vi "ResultsGui.FindFiles.vi"(6 "File content prev":T1[](array[typedef]), 7 "File list tree":refnum<vi>, 8 "error in (no error)":errorcluster, 9 "PageSize (100)":i32=100, 10 "PageIdx":i32, 11 "Paths":path[](array[path])) -> (0 "error out":errorcluster, 2 "File content":T1[](array[typedef]), 3 "TotalSize":i32)   [LabVIEW 2016]
uses:
  Logger/Logger.File.ctl
  Logger/Logger.File.Properties.ctl
  Sequence/Sequence.Code.SerialFormat.ctl
  Sequence/Sequence.Counters.ctl
  Logger/Logger.File.Serials.ctl
  Sequence/Sequence.Step.Status.ctl
  <vilib>/Utility/miscctls.llb/LVRowAndColumnTypeDef.ctl
  <vilib>/Utility/miscctls.llb/LVNodeAndColumnTypeDef.ctl
  tools/Translator/Translator.Message.ctl
  tools/Translator/Translator.FormatMessage.vi
  tools/Translator/Translator.Global.vi
  Global/ApplicationGlobal.vi
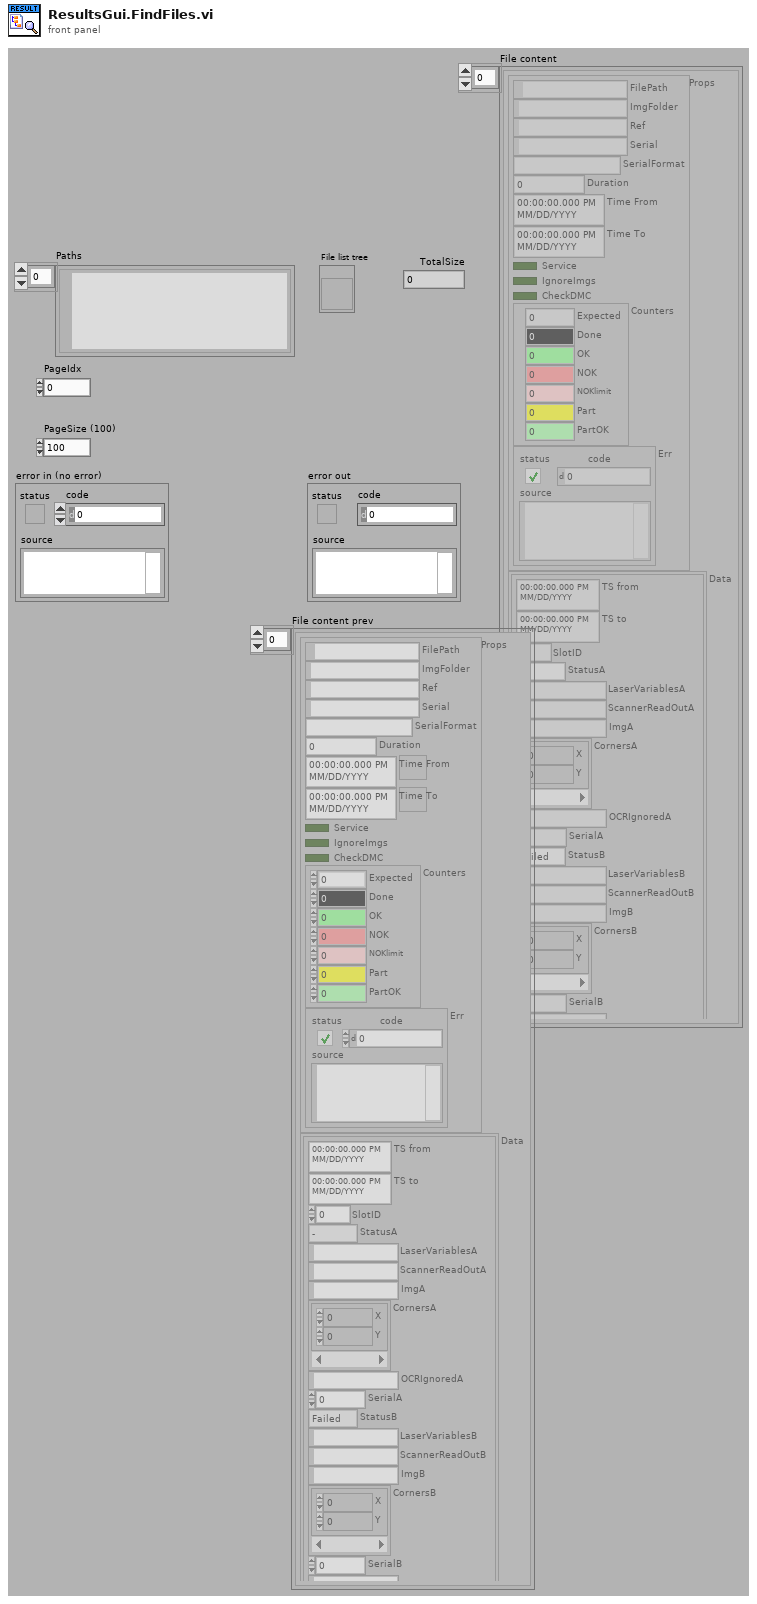
[diagram p1: front panel]
types:
  T1 = typedef "Logger.File.ctl" = cluster{"Props":T2, "Data":T5[]}
  T2 = typedef "Logger.File.Properties.ctl" = cluster{"FilePath":path, "ImgFolder":string, "Ref":string, "Serial":string, "SerialFormat":T3, "Duration":dbl, "Time From":timestamp, "Time To":timestamp, "Service":bool, "IgnoreImgs":bool, "CheckDMC":bool, "Counters":T4, "Err":errorcluster}
  T3 = typedef "Sequence.Code.SerialFormat.ctl" = enum8{"", "6 dig", "7 dig"}
  T4 = typedef "Sequence.Counters.ctl" = cluster{"Expected":u16, "Done":u16, "OK":u16, "NOK":u16, "NOKlimit":u16, "Part":u16, "PartOK":u16}
  T5 = typedef "Logger.File.Serials.ctl" = cluster{"TS from":timestamp, "TS to":timestamp, "SlotID":u8, "StatusA":T6, "LaserVariablesA":string, "ScannerReadOutA":string, "ImgA":string, "CornersA":cluster{"X":i32, "Y":i32}[], "OCRIgnoredA":string, "SerialA":u8, "StatusB":T6, "LaserVariablesB":string, "ScannerReadOutB":string, "ImgB":string, "CornersB":cluster{"X":i32, "Y":i32}[], "SerialB":u8, "OCRIgnoredB":string}
  T6 = typedef "Sequence.Step.Status.ctl" = enum16{"-", "Pending", "Running", "Skipped", "Passed", "Failed", "Done", "Error", "Aborted", "Stopped"}
  T7 = typedef "Translator.Message.ctl" = enum16{"-", "Event confirmed", "Log out", "Log in", "Shutdown", "Cancel", "Start", "Begin time", "End time", "Duration", "Service Mode", "Ignore Results", "Serial Format", "On", "Off", "OK", "NOK", "NOK %s", "Home", "Work", "Close", "Open", "In progress...", "Missing", "Empty", "Hardware failure", "Initial", "Default", "Total", "Out of range", "Free disk space is below 1GB - contact technician", "Error %d >> %s", "Error %d >> %s >> %s", "Msg %d >> %s", "Laser msg %d %s", "Laser cmd error %s %d", "Laser cmd failed %s", "Laser cmd warning %s", "Laser disconnected", "Laser status %s", "Laser already started", "Laser job unkonwn %s", "Laser job missing %s", "Laser job select failure %s", "Unable to start laser printing (%s)", "Unable to stop laser printing (%s)", "Laser marking aborted", "Laser marking timeout", "Unable to reset Laser Interlock (%s)", "Unable to trigger Laser. Laser not ready (%s)", "Laser job '%s' coordinates not configured", "Starting %s", "Quitting %s", "Configured", "Initializing", "Quitting", "Loading", "Loaded %d results", "Loaded %d events", "Running", "Stopped", "Summary", "Laser", "Do you want to continue?", "Do you want to delete the configuration?", "The configuration is being used by an order. Unable to delete!", "Press confirm button", "Station is not based. Do you want to exit?", "Station requires changeover. Do you want to run the test?", "Test options are not set as default. Do you want to continue?", "Formatting of WabcoNo is disabled. Do you want to continue?", "Product not detected. Do you want to continue?", "Product scan failed. Do you want to continue?", "Calibration", "Log out?", "System", "All", "IDLE", "Translating...%s", "Not found", "Alarm %s", "Run", "Skip", "Abort", "Repeat", "Please wait...", "Database disconnected", "Database disconnected - changeover disabled!", "Login to database successful", "Login to database failed: %d; %s", "Unable to check the product status of reference %d - database disconnected", "Unable to set the product status of reference %d - database disconnected", "Variant file backup %s", "Read variant (%s)", "Result", "Station armed!", "Station requires changeover!", "Select reference number...", "EMERGENCY BUTTON - press Control button", "EMERGENCY DOOR - press Control button", "Resetting Emergency...", "Unable to reset safety circuit - Emergency Button pressed", "Unable to reset safety circuit - Emergency Side Door open", "Station not based", "Station based", "Station not empty", "Station basing...", "No order", "Press Start to begin new order", "Scanning new order", "Order NOK. Correct or scan again", "Order OK. Press Accept", "Order ready", "Revolver incorrect", "Fork incorrect", "Revolver missing", "Revolver empty", "Container missing", "Offline results", "Offline statistics", "Updating statistics %.1f %%", "DMC Configurator", "Door open", "Close the front door", "Press start button", "Done. Open the front door", "Running...", "Running...%.1f %%", "Pause %s", "Pause %s. NOK container missing", "Pause %s. OK container missing", "Pause %s. Revolver empty", "Pause %s. Revolver missing", "Pause %s. Revolver incorrect", "Pause %s. Fork missing", "Pause %s. Fork incorrect", "Pause %s. Too many failures", "Pause %s. Unloading failure", "Pause %s. One slot is not working", "Pause %s. Part order is done. Empty OK container", "Pause %s. Unable to move product to slot", "Pause %s. Unable to move back product pusher", "Pause %s. Unable to lift product", "Pause %s. Unable to move back product lifter", "Pause %s. Unable to move product arm to Work", "Pause %s. Unable to move product arm to NOK", "Pause %s. Unable to move product arm to OK", "Pause %s. Unable to unsuck the NOK product", "Pause %s. Unable to drop the NOK product", "Pause %s. Product OK missing", "Pause %s. Unable to unsuck the OK product", "Pause %s. Unable to drop the OK product", "Stopping...", "File '%s' is missing", "File '%s' is broken", "File '%s' is running", "Log file started (%s)", "Log file ended (%s)", "Log file stopped (%s)", "Log file ignored (%s)", "Log file exported (%s)", "Log file export failed (%s)", "Wrong serial number in log file", "Wrong reference number in log file", "Test steps are missing", "%s = %.3f", "Process param '%s' not found in DB", "Process param '%s' wrong order", "Process param '%s' value %.3f out of limits (%.3f; %.3f)", "Step%d param '%s' not found in DB", "Step%d param '%s' wrong order", "Step%d param '%s' value %.3f out of limits (%.3f; %.3f)", "Step%d EV '%s' not found in DB", "Step%d EV '%s' wrong order", "\"%s\" not found in DB", "\"%s\" wrong order", "\"%s\" value %.3f out of limits (%.3f; %.3f)", "\"%s\" not found in software", "Process init (%s)", "Process started", "Process restarted", "Process run", "Process done", "Process done - remove OK container", "Process aborted", "Process aborted at work", "Process aborted at home", "Process error", "Process error at home", "Process error at work", "Process close", "Process pause", "Process continue", "Process door open", "Process door close", "Process pause at slot %s due to %s", "Select plate from the order to process", "Do you want to start the process?", "Do you want to continue the process?", "There is unfinished order. Do you want to put the new order?", "Product %s %d OK", "Product %s %d NOK", "Unable to unload the slot %s. Product missing in the slot", "Unable to unload the slot %s. Product already in the arm", "Unable to accept the product as OK. Product missing in slot %s", "Unable to accept the product as OK. Product could not drop into the container at slot %s", "Unable to accept the product as NOK. Product could not drop into the container at slot %s", "Scan failed. Error %s", "Scan failed. Scanner disconnected", "Scan failed. Wrong Wabco number %d, limit (%d,%d)", "Scan failed. Wrong serial number %d, limit (%d,%d)", "Scan failed. Wrong date %d, limit (%d,%d)", "Scan failed. Wrong product wabco number %d (expected %d)", "Scan failed. Wrong product serial number %d (expected > 0)", "Scan OK %s", "Scan failed. Unable to determine table position (%s)", "Scan failed. Timeout", "Tune failed. Scanner disconnected", "Tune failed. Timeout", "%s = %d", "%s = %d->%d", "Unable to set %s = %.2f - Air Pressure Inside off", "Unable to set digital output '%s' = %d", "Unable to activate air pressure inside - timeout", "Unable to activate air pressure inside - aborted", "Unable to switch on Air Main Valve - Air Pressure Inlet off", "Unable to switch on Air Main Valve - Door open", "Unable to switch off Air Main Valve - timeout", "Unable to switch off Air Main Valve - aborted", "Unable to rotate Table - timeout", "Unable to rotate Table - aborted", "Unable to rotate Table - Product Move not in Home position", "Unable to rotate Table - Air Pressure Inside off", "Unable to rotate Table - Product Lift A not in Home position", "Unable to rotate Table - Product Lift B not in Home position", "Unable to rotate Table - unlock before movement timeout", "Unable to rotate Table - lock after movement timeout", "Unable to move Table Lock to %s position - timeout", "Unable to move Table Lock to %s position - aborted", "Unable to move Table Lock to %s position - Air Pressure Inside off", "Unable to move Table Lock to %s position - Table not in position", "Unable to move Product Lift A to %s position - timeout", "Unable to move Product Lift B to %s position - timeout", "Unable to move Product Lift A to %s position - aborted", "Unable to move Product Lift B to %s position - aborted", "Unable to move Product Lift A to %s position - Air Pressure Inside off", "Unable to move Product Lift B to %s position - Air Pressure Inside off", "Unable to move Product Lift A to %s position - Table not locked", "Unable to move Product Lift B to %s position - Table not locked", "Unable to move Product Lift A to %s position - Product Arm not in Work position", "Unable to move Product Lift B to %s position - Product Arm not in Work position", "Unable to set Product Suction Gripper %s to %s - timeout", "Unable to set Product Suction Gripper %s to %s - aborted", "Unable to set Product Suction Gripper %s to %s - Air Pressure Inside off", "Unable to set Product Suction Gripper %s to %s - Table slot unkown", "Unable to move Product Arm to %s position - timeout", "Unable to move Product Arm to %s position - aborted", "Unable to move Product Arm to %s position - Air Pressure Inside off", "Unable to move Product Arm to %s position - Product Lift A not in Home position", "Unable to move Product Arm to %s position - Product Lift B not in Home position", "Unable to move Product to %s position - timeout", "Unable to move Product to %s position - aborted", "Unable to move Product to %s position - Air Pressure Inside off", "Unable to move Product to %s position - Table not in position"}
  T8 = typedef "LVNodeAndColumnTypeDef.ctl" = cluster{"Node":string, "Column":i32}
  T9 = typedef "LVRowAndColumnTypeDef.ctl" = cluster{"Row":i32, "Column":i32}
  T10 = cluster{"last mod":timestamp, "appended path":path}
  T11 = cluster{"last mod":timestamp, "appended path":path}[]
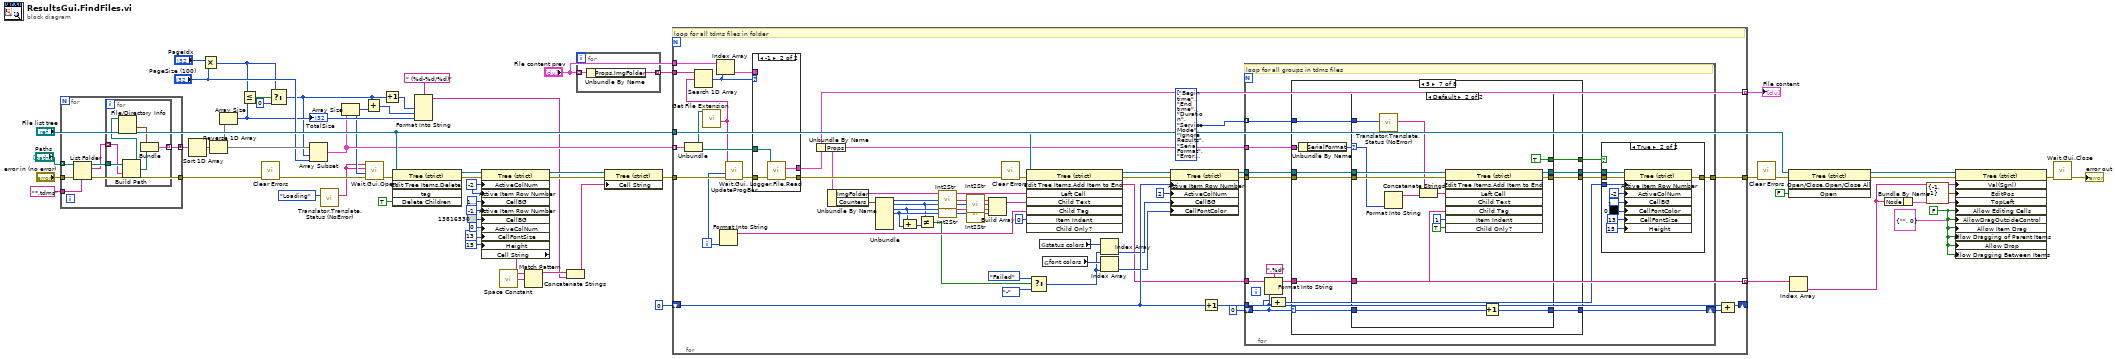
[diagram p0: block diagram]
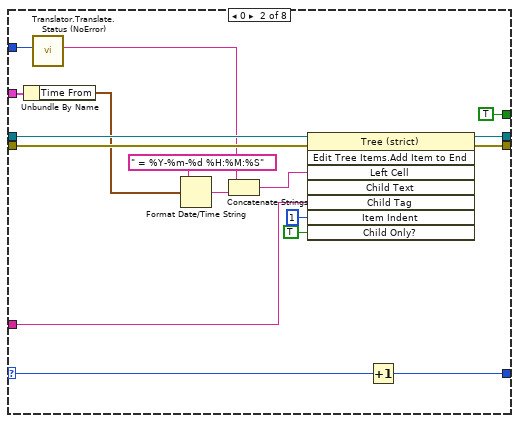
[diagram p5: hidden frame]
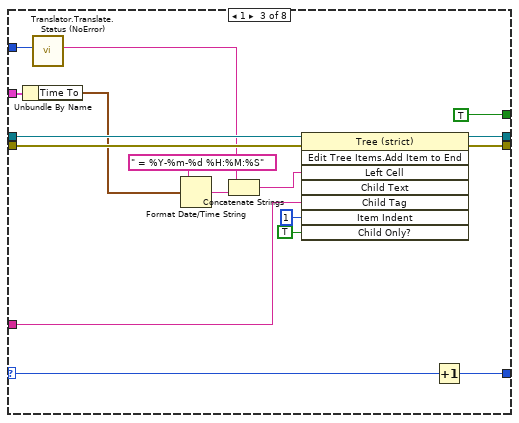
[diagram p6: hidden frame]
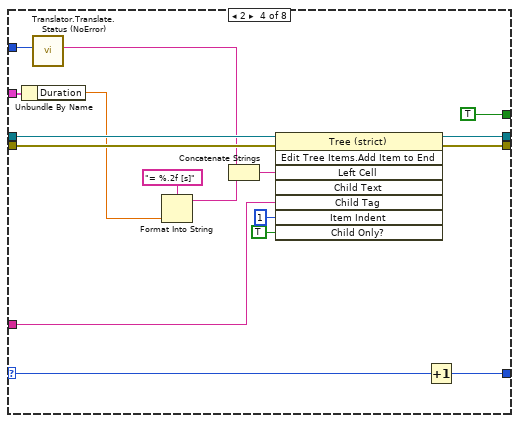
[diagram p7: hidden frame]
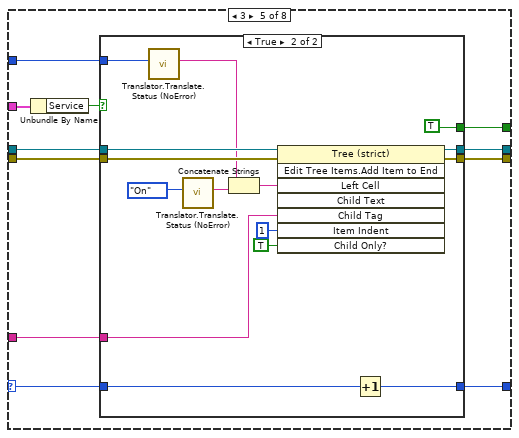
[diagram p8: hidden frame]
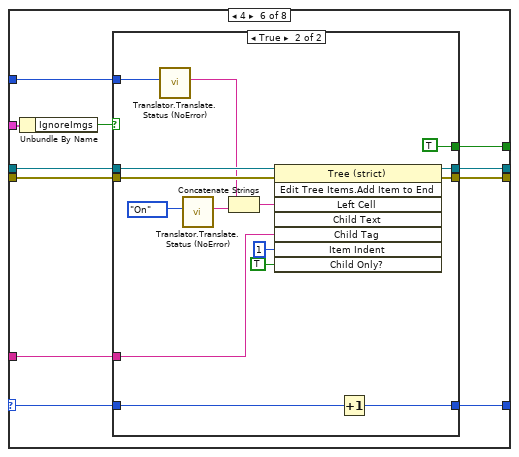
[diagram p10: hidden frame]
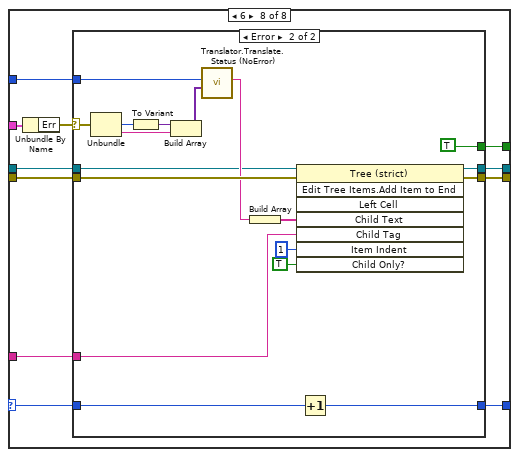
[diagram p13: hidden frame]
diagram:
  w41 = -2 ("Active Cell:Active Column Number")
  w54 = FALSE ("Allow Editing Cells")
  n1 = for {
    tunnel: "*.tdms" ("pattern") -> [w65]
    tunnel: "Paths" -> [w64] mode=indexing
    tunnel: [w61] -> w43 mode=concatenating
    tunnel: "error in (no error)" -> [w66]
    tunnel: [w62] -> w48
    n2 = List Folder(path=w64, pattern=w65, error in=w66) -> (path out=w63:path, filenames=w60:string[], error out=w62:errorcluster)  [unwired: 1 in, 1 out]
    n3 = for {
      tunnel: w60 -> [w69] mode=indexing
      tunnel: w63 -> [w71]
      tunnel: [w70] -> w61 mode=indexing
      n4 = Build Path(base path=w71, name or relative path=w69) -> (appended path=w68:path)
      n5 = File/Directory Info(path=w68) -> (last mod=w67:timestamp)  [unwired: 1 in, 6 out]
      n6 = Bundle("last mod"=w67, "appended path"=w68) -> (w70:T10)  [unwired: 1 in]
    }
  }
  n7 = Sort 1D Array(array=w43) -> (sorted array=w57:T11)
  n8 = Multiply(x="PageIdx", y="PageSize (100)") -> (x*y=w29:i32)
  n9 = Reverse 1D Array(array=w57) -> (reversed array=w32:T11)
  n10 = Array Size(array=w32) -> (size(s)=w23:i32)
  "TotalSize" <- w23
  n11 = Less Or Equal?(x=w29, y=w23) -> (x <= y?=w30:bool)
  n12 = call <vilib>:"Clear Errors.vi"("error in (no error)"=w48) -> ("error out"=w13:errorcluster)  [unwired: 5 in, 1 out]
  n13 = Select(t=w29, s=w30, f=0) -> (s? t:f=w18:i32)
  n14 = Array Subset(array=w32, index=w18, length="PageSize (100)") -> (w19:T11)
  n15 = call "Translator.Translate.Status (NoError).vi"("msg"=Translator.Message."Loading") -> ("Translated Msg"=w9:string)  [unwired: 10 in]
  n16 = Array Size(array=w19) -> (size(s)=w11:i32)
  n17 = Add(x=w18, y=w11) -> (x+y=w17:i32)
  n18 = call "Wait.Gui.Open.vi"("error in (no error)"=w13, "ProgBarSize (0)"=w11, "Status (\"\")"=w9, "Msg"=w9) -> ("error out"=w12:errorcluster)  [unwired: 7 in]
  n19 = Increment(x=w18) -> (x+1=w16:i32)
  n20 = invoke on="Invoke Node" class="Tree (strict)" method="Edit Tree Items.Delete"(reference="File list tree", error in=w12, "Delete Children"=TRUE ("Delete Children?")) -> (reference out=w38:refnum<vi>, error out=w37:errorcluster)  [unwired: 2 in, 3 out]
  n21 = Format Into String(format string=" (%d-%d/%d)", w16, w17, w23) -> (resulting string=w3:string)  [unwired: 2 in, 1 out]
  n22 = property on="Property Node" class="Tree (strict)"(reference=w38, error in=w37, "ActiveColNum"=w41, "Active Item Row Number"=w41, "CellBG"=u32 16777225, "Active Item Row Number"=-1 ("Active Item:Row Number"), "CellBG"=u32 13816530, "ActiveColNum"=0 ("Active Cell:Active Column Number"), "CellFontSize"=u32 13 ("Active Cell:Cell Font:Size"), "Height"=15 ("Active Cell:Cell Size:Height")) -> (reference out=w26:refnum<vi>, error out=w27:errorcluster, "Cell String"=w4:string)
  n23 = call <vilib>:"Space Constant.vi"() -> ("String"=w24:string)
  n24 = Match Pattern(string=w4, regular expression=w24) -> (before substring=w21:string)  [unwired: 1 in, 3 out]
  n25 = Concatenate Strings(w21, w3) -> (w20:string)
  n26 = for {
    tunnel: "File content prev" -> [w73] mode=indexing
    tunnel: [w72] -> w8 mode=indexing
    n27 = Unbundle By Name(w73) -> ("Props.ImgFolder"=w72:string)
  }
  n28 = property on="Property Node" class="Tree (strict)"(reference=w26, error in=w27, "Cell String"=w20) -> (error out=w25:errorcluster)  [unwired: 1 out]
  n29 = for {
    tunnel: "File list tree" -> [w104]
    tunnel: [w98] -> w46 mode=indexing
    tunnel: [w121] -> w45 mode=indexing
    tunnel: w19 -> [w118] mode=indexing
    shift-right: [w82] -> _
    shift-left: 0 -> [w114]
    tunnel: w25 -> [w123]
    tunnel: [w105] -> w52
    tunnel: w8 -> [w103]
    tunnel: "File content prev" -> [w102]
    i -> [w106]
    w87 = T7[] [enum."Begin time", enum."End time", enum."Duration", enum."Service Mode", enum."Ignore Results", enum."Serial Format", enum."Error %d >> %s"] items=["-", "Event confirmed", "Log out", "Log in", "Shutdown", "Cancel", "Start", "Begin time", "End time", "Duration", "Service Mode", "Ignore Results", "Serial Format", "On", "Off", "OK", "NOK", "NOK %s", "Home", "Work", "Close", "Open", "In progress...", "Missing", "Empty", "Hardware failure", "Initial", "Default", "Total", "Out of range", "Free disk space is below 1GB - contact technician", "Error %d >> %s", "Error %d >> %s >> %s", "Msg %d >> %s", "Laser msg %d %s", "Laser cmd error %s %d", "Laser cmd failed %s", "Laser cmd warning %s", "Laser disconnected", "Laser status %s", "Laser already started", "Laser job unkonwn %s", "Laser job missing %s", "Laser job select failure %s", "Unable to start laser printing (%s)", "Unable to stop laser printing (%s)", "Laser marking aborted", "Laser marking timeout", "Unable to reset Laser Interlock (%s)", "Unable to trigger Laser. Laser not ready (%s)", "Laser job '%s' coordinates not configured", "Starting %s", "Quitting %s", "Configured", "Initializing", "Quitting", "Loading", "Loaded %d results", "Loaded %d events", "Running", "Stopped", "Summary", "Laser", "Do you want to continue?", "Do you want to delete the configuration?", "The configuration is being used by an order. Unable to delete!", "Press confirm button", "Station is not based. Do you want to exit?", "Station requires changeover. Do you want to run the test?", "Test options are not set as default. Do you want to continue?", "Formatting of WabcoNo is disabled. Do you want to continue?", "Product not detected. Do you want to continue?", "Product scan failed. Do you want to continue?", "Calibration", "Log out?", "System", "All", "IDLE", "Translating...%s", "Not found", "Alarm %s", "Run", "Skip", "Abort", "Repeat", "Please wait...", "Database disconnected", "Database disconnected - changeover disabled!", "Login to database successful", "Login to database failed: %d; %s", "Unable to check the product status of reference %d - database disconnected", "Unable to set the product status of reference %d - database disconnected", "Variant file backup %s", "Read variant (%s)", "Result", "Station armed!", "Station requires changeover!", "Select reference number...", "EMERGENCY BUTTON - press Control button", "EMERGENCY DOOR - press Control button", "Resetting Emergency...", "Unable to reset safety circuit - Emergency Button pressed", "Unable to reset safety circuit - Emergency Side Door open", "Station not based", "Station based", "Station not empty", "Station basing...", "No order", "Press Start to begin new order", "Scanning new order", "Order NOK. Correct or scan again", "Order OK. Press Accept", "Order ready", "Revolver incorrect", "Fork incorrect", "Revolver missing", "Revolver empty", "Container missing", "Offline results", "Offline statistics", "Updating statistics %.1f %%", "DMC Configurator", "Door open", "Close the front door", "Press start button", "Done. Open the front door", "Running...", "Running...%.1f %%", "Pause %s", "Pause %s. NOK container missing", "Pause %s. OK container missing", "Pause %s. Revolver empty", "Pause %s. Revolver missing", "Pause %s. Revolver incorrect", "Pause %s. Fork missing", "Pause %s. Fork incorrect", "Pause %s. Too many failures", "Pause %s. Unloading failure", "Pause %s. One slot is not working", "Pause %s. Part order is done. Empty OK container", "Pause %s. Unable to move product to slot", "Pause %s. Unable to move back product pusher", "Pause %s. Unable to lift product", "Pause %s. Unable to move back product lifter", "Pause %s. Unable to move product arm to Work", "Pause %s. Unable to move product arm to NOK", "Pause %s. Unable to move product arm to OK", "Pause %s. Unable to unsuck the NOK product", "Pause %s. Unable to drop the NOK product", "Pause %s. Product OK missing", "Pause %s. Unable to unsuck the OK product", "Pause %s. Unable to drop the OK product", "Stopping...", "File '%s' is missing", "File '%s' is broken", "File '%s' is running", "Log file started (%s)", "Log file ended (%s)", "Log file stopped (%s)", "Log file ignored (%s)", "Log file exported (%s)", "Log file export failed (%s)", "Wrong serial number in log file", "Wrong reference number in log file", "Test steps are missing", "%s = %.3f", "Process param '%s' not found in DB", "Process param '%s' wrong order", "Process param '%s' value %.3f out of limits (%.3f; %.3f)", "Step%d param '%s' not found in DB", "Step%d param '%s' wrong order", "Step%d param '%s' value %.3f out of limits (%.3f; %.3f)", "Step%d EV '%s' not found in DB", "Step%d EV '%s' wrong order", "\"%s\" not found in DB", "\"%s\" wrong order", "\"%s\" value %.3f out of limits (%.3f; %.3f)", "\"%s\" not found in software", "Process init (%s)", "Process started", "Process restarted", "Process run", "Process done", "Process done - remove OK container", "Process aborted", "Process aborted at work", "Process aborted at home", "Process error", "Process error at home", "Process error at work", "Process close", "Process pause", "Process continue", "Process door open", "Process door close", "Process pause at slot %s due to %s", "Select plate from the order to process", "Do you want to start the process?", "Do you want to continue the process?", "There is unfinished order. Do you want to put the new order?", "Product %s %d OK", "Product %s %d NOK", "Unable to unload the slot %s. Product missing in the slot", "Unable to unload the slot %s. Product already in the arm", "Unable to accept the product as OK. Product missing in slot %s", "Unable to accept the product as OK. Product could not drop into the container at slot %s", "Unable to accept the product as NOK. Product could not drop into the container at slot %s", "Scan failed. Error %s", "Scan failed. Scanner disconnected", "Scan failed. Wrong Wabco number %d, limit (%d,%d)", "Scan failed. Wrong serial number %d, limit (%d,%d)", "Scan failed. Wrong date %d, limit (%d,%d)", "Scan failed. Wrong product wabco number %d (expected %d)", "Scan failed. Wrong product serial number %d (expected > 0)", "Scan OK %s", "Scan failed. Unable to determine table position (%s)", "Scan failed. Timeout", "Tune failed. Scanner disconnected", "Tune failed. Timeout", "%s = %d", "%s = %d->%d", "Unable to set %s = %.2f - Air Pressure Inside off", "Unable to set digital output '%s' = %d", "Unable to activate air pressure inside - timeout", "Unable to activate air pressure inside - aborted", "Unable to switch on Air Main Valve - Air Pressure Inlet off", "Unable to switch on Air Main Valve - Door open", "Unable to switch off Air Main Valve - timeout", "Unable to switch off Air Main Valve - aborted", "Unable to rotate Table - timeout", "Unable to rotate Table - aborted", "Unable to rotate Table - Product Move not in Home position", "Unable to rotate Table - Air Pressure Inside off", "Unable to rotate Table - Product Lift A not in Home position", "Unable to rotate Table - Product Lift B not in Home position", "Unable to rotate Table - unlock before movement timeout", "Unable to rotate Table - lock after movement timeout", "Unable to move Table Lock to %s position - timeout", "Unable to move Table Lock to %s position - aborted", "Unable to move Table Lock to %s position - Air Pressure Inside off", "Unable to move Table Lock to %s position - Table not in position", "Unable to move Product Lift A to %s position - timeout", "Unable to move Product Lift B to %s position - timeout", "Unable to move Product Lift A to %s position - aborted", "Unable to move Product Lift B to %s position - aborted", "Unable to move Product Lift A to %s position - Air Pressure Inside off", "Unable to move Product Lift B to %s position - Air Pressure Inside off", "Unable to move Product Lift A to %s position - Table not locked", "Unable to move Product Lift B to %s position - Table not locked", "Unable to move Product Lift A to %s position - Product Arm not in Work position", "Unable to move Product Lift B to %s position - Product Arm not in Work position", "Unable to set Product Suction Gripper %s to %s - timeout", "Unable to set Product Suction Gripper %s to %s - aborted", "Unable to set Product Suction Gripper %s to %s - Air Pressure Inside off", "Unable to set Product Suction Gripper %s to %s - Table slot unkown", "Unable to move Product Arm to %s position - timeout", "Unable to move Product Arm to %s position - aborted", "Unable to move Product Arm to %s position - Air Pressure Inside off", "Unable to move Product Arm to %s position - Product Lift A not in Home position", "Unable to move Product Arm to %s position - Product Lift B not in Home position", "Unable to move Product to %s position - timeout", "Unable to move Product to %s position - aborted", "Unable to move Product to %s position - Air Pressure Inside off", "Unable to move Product to %s position - Table not in position"]
    # "loop for all tdms files in folder"
    n30 = Unbundle(w118) -> ("appended path"=w99:path)  [unwired: 1 out]
    n31 = call <vilib>:"Get File Extension.vi"("file"=w99) -> ("filename without extension"=w89:string)  [unwired: 6 in, 4 out]
    n32 = Search 1D Array(1D array=w103, element=w89) -> (index of element=w101:i32)  [unwired: 1 in]
    n33 = Index Array(array=w102, index=w101) -> (element=w100:T1)
    n34 = Format Into String(w106) -> (resulting string=w120:string)  [unwired: 3 in, 1 out]
    n35 = call "Wait.Gui.UpdateProgBar.vi"("error in (no error)"=w123, "ProgBar (0)"=w106, "status (\"\")"=w89) -> ("error out"=w107:errorcluster)  [unwired: 8 in]
    n36 = case shown="-1" w101 {
      tunnel: [w125 w129] -> w122
      tunnel: [w124 w128] -> w121
      tunnel: w99 -> [_ w127]
      tunnel: w107 -> [w125 w126]
      tunnel: w100 -> [w124 _]
      frame Default {
      }
      frame -1 {
        n37 = call "Logger.File.Read.vi"("error in (no error)"=w126, "file path"=w127) -> ("error out"=w129:errorcluster, "File content"=w128:T1)  [unwired: 6 in, 2 out]
      }
    }
    n38 = Unbundle By Name(w121) -> ("Props"=w88:T2)
    n39 = Unbundle By Name(w88) -> ("ImgFolder"=w97:string, "Counters"=w95:T4)
    n40 = Unbundle(w95) -> ("Expected"=w96:u16, "Done"=w78:u16, "OK"=w80:u16, "NOK"=w81:u16)  [unwired: 3 out]
    n41 = Compound Arithmetic op=ADD(w80, w81) -> (w79:u16)
    n42 = Not Equal?(x=w78, y=w79) -> (x != y?=w77:bool)
    n43 = call "Int2Str.vi"("Numeric"=w96) -> ("string"=w93:string)
    n44 = call "Int2Str.vi"("Numeric"=w80) -> ("string"=w92:string)
    n45 = call "Int2Str.vi"("Numeric"=w78) -> ("string"=w94:string)
    n46 = call "Int2Str.vi"("Numeric"=w81) -> ("string"=w91:string)
    n47 = Build Array(w93, w94, w92, w91) -> (w90:string[])
    n48 = call <vilib>:"Clear Errors.vi"("error in (no error)"=w122) -> ("error out"=w111:errorcluster)  [unwired: 5 in, 1 out]
    n49 = invoke on="Invoke Node" class="Tree (strict)" method="Edit Tree Items.Add Item to End"(reference=w104, error in=w111, "Left Cell"=w97, "Child Text"=w90, "Child Tag"=w120, "Item Indent"=0 ("New Item Indentation")) -> (reference out=w116:refnum<vi>, error out=w117:errorcluster, "Edit Tree Items:Add Item to End"=w98:string)  [unwired: 2 in, 5 out]
    n50 = Select(t=Sequence.Step.Status."Failed" ("Status"), s=w77, f=Sequence.Step.Status."-" ("Status")) -> (s? t:f=w74:T6)
    n51 = global read "ApplicationGlobal.vi" "status colors"() -> (w112:u32[])
    n52 = global read "ApplicationGlobal.vi" "font colors"() -> (w110:u32[])
    n53 = Index Array(array=w112, index=w74) -> (element=w109:u32)
    n54 = Index Array(array=w110, index=w74) -> (element=w108:u32)
    n55 = property on="Property Node" class="Tree (strict)"(reference=w116, error in=w117, "Active Item Row Number"=w114, "ActiveColNum"=2 ("Active Cell:Active Column Number"), "CellBG"=w109, "CellFontColor"=w108) -> (reference out=w84:refnum<vi>, error out=w115:errorcluster)
    n56 = Increment(x=w114) -> (x+1=w83:i32)
    n57 = for {
      tunnel: w84 -> [w143]
      tunnel: w98 -> [w142]
      tunnel: w115 -> [w144]
      tunnel: [w131] -> w105
      tunnel: w88 -> [w139]
      tunnel: w87 -> [w138] mode=indexing
      shift-right: [w137] -> w85
      shift-left: 0 -> [w136]
      tunnel: w83 -> [w135]
      # "loop for all groups in tdms files"
      n58 = Format Into String(format string=".%d", initial string=w142, w136) -> (resulting string=w140:string)  [unwired: 1 in, 1 out]
      n59 = Compound Arithmetic op=ADD(w135, w136) -> (w134:i32)
      n60 = case shown="5" w136 {
        selector: w136 -> [w156 w162 w179 w196 w213 w242 w271 w298]
        tunnel: w144 -> [w157 w174 w191 w208 w219 w248 w277 w302]
        tunnel: w143 -> [w155 w173 w190 w207 w218 w247 w276 w299]
        tunnel: w140 -> [_ w172 w189 w206 w217 w246 w275 w300]
        tunnel: [w157 w169 w186 w203 w216 w245 w274 w301] -> w132
        tunnel: w139 -> [_ w167 w184 w202 w215 w244 w273 w305]
        tunnel: w138 -> [_ w166 w183 w201 w211 w240 w269 w306]
        tunnel: [w156 w161 w178 w197 w212 w241 w270 w303] -> w137
        tunnel: [w155 w159 w176 w193 w210 w239 w268 w297] -> w133
        tunnel: [_ TRUE TRUE TRUE w209 w238 w267 w296] -> w130
        frame Default {
        }
        frame 0 {
          n61 = Unbundle By Name(w167) -> ("Time From"=w168:timestamp)
          n62 = call "Translator.Translate.Status (NoError).vi"("msg"=w166) -> ("Translated Msg"=w164:string)  [unwired: 10 in]
          n63 = Format Date/Time String(time format string (%c)=" = %Y-%m-%d %H:%M:%S", seconds (now)=w168) -> (date/time string=w165:string)  [unwired: 1 in]
          n64 = Concatenate Strings(w164, w165) -> (w160:string)
          n65 = invoke on="Invoke Node" class="Tree (strict)" method="Edit Tree Items.Add Item to End"(reference=w173, error in=w174, "Left Cell"=w160, "Child Tag"=w172, "Item Indent"=1 ("New Item Indentation"), "Child Only?"=TRUE) -> (reference out=w159:refnum<vi>, error out=w169:errorcluster)  [unwired: 2 in, 6 out]
          n66 = Increment(x=w162) -> (x+1=w161:i32)
        }
        frame 1 {
          n67 = Unbundle By Name(w184) -> ("Time To"=w185:timestamp)
          n68 = call "Translator.Translate.Status (NoError).vi"("msg"=w183) -> ("Translated Msg"=w181:string)  [unwired: 10 in]
          n69 = Format Date/Time String(time format string (%c)=" = %Y-%m-%d %H:%M:%S", seconds (now)=w185) -> (date/time string=w182:string)  [unwired: 1 in]
          n70 = Concatenate Strings(w181, w182) -> (w177:string)
          n71 = invoke on="Invoke Node" class="Tree (strict)" method="Edit Tree Items.Add Item to End"(reference=w190, error in=w191, "Left Cell"=w177, "Child Tag"=w189, "Item Indent"=1 ("New Item Indentation"), "Child Only?"=TRUE) -> (reference out=w176:refnum<vi>, error out=w186:errorcluster)  [unwired: 2 in, 6 out]
          n72 = Increment(x=w179) -> (x+1=w178:i32)
        }
        frame 2 {
          n73 = Unbundle By Name(w202) -> ("Duration"=w199:dbl)
          n74 = call "Translator.Translate.Status (NoError).vi"("msg"=w201) -> ("Translated Msg"=w200:string)  [unwired: 10 in]
          n75 = Format Into String(format string="= %.2f [s]", w199) -> (resulting string=w194:string)  [unwired: 2 in, 1 out]
          n76 = Concatenate Strings(w200, w194) -> (w195:string)
          n77 = invoke on="Invoke Node" class="Tree (strict)" method="Edit Tree Items.Add Item to End"(reference=w207, error in=w208, "Left Cell"=w195, "Child Tag"=w206, "Item Indent"=1 ("New Item Indentation"), "Child Only?"=TRUE) -> (reference out=w193:refnum<vi>, error out=w203:errorcluster)  [unwired: 2 in, 6 out]
          n78 = Increment(x=w196) -> (x+1=w197:i32)
        }
        frame 3 {
          n79 = Unbundle By Name(w215) -> ("Service"=w214:bool)
          n80 = case shown="True" w214 {
            tunnel: w219 -> [w222 w237]
            tunnel: w218 -> [w220 w236]
            tunnel: w217 -> [_ w235]
            tunnel: [w222 w232] -> w216
            tunnel: w211 -> [_ w227]
            tunnel: w213 -> [w221 w231]
            tunnel: [w221 w230] -> w212
            tunnel: [w220 w224] -> w210
            tunnel: [_ TRUE] -> w209
            frame False {
            }
            frame True {
              n81 = call "Translator.Translate.Status (NoError).vi"("msg"=w227) -> ("Translated Msg"=w226:string)  [unwired: 10 in]
              n82 = call "Translator.Translate.Status (NoError).vi"("msg"=Translator.Message."On") -> ("Translated Msg"=w228:string)  [unwired: 10 in]
              n83 = Concatenate Strings(w226, w228) -> (w225:string)
              n84 = invoke on="Invoke Node" class="Tree (strict)" method="Edit Tree Items.Add Item to End"(reference=w236, error in=w237, "Left Cell"=w225, "Child Tag"=w235, "Item Indent"=1 ("New Item Indentation"), "Child Only?"=TRUE) -> (reference out=w224:refnum<vi>, error out=w232:errorcluster)  [unwired: 2 in, 6 out]
              n85 = Increment(x=w231) -> (x+1=w230:i32)
            }
          }
        }
        frame 4 {
          n86 = Unbundle By Name(w244) -> ("IgnoreImgs"=w243:bool)
          n87 = case shown="True" w243 {
            tunnel: w248 -> [w251 w266]
            tunnel: w247 -> [w249 w265]
            tunnel: w246 -> [_ w264]
            tunnel: [w251 w254] -> w245
            tunnel: w242 -> [w250 w261]
            tunnel: [w250 w260] -> w241
            tunnel: w240 -> [_ w257]
            tunnel: [w249 w253] -> w239
            tunnel: [_ TRUE] -> w238
            frame False {
            }
            frame True {
              n88 = call "Translator.Translate.Status (NoError).vi"("msg"=w257) -> ("Translated Msg"=w256:string)  [unwired: 10 in]
              n89 = call "Translator.Translate.Status (NoError).vi"("msg"=Translator.Message."On") -> ("Translated Msg"=w258:string)  [unwired: 10 in]
              n90 = Concatenate Strings(w256, w258) -> (w255:string)
              n91 = invoke on="Invoke Node" class="Tree (strict)" method="Edit Tree Items.Add Item to End"(reference=w265, error in=w266, "Left Cell"=w255, "Child Tag"=w264, "Item Indent"=1 ("New Item Indentation"), "Child Only?"=TRUE) -> (reference out=w253:refnum<vi>, error out=w254:errorcluster)  [unwired: 2 in, 6 out]
              n92 = Increment(x=w261) -> (x+1=w260:i32)
            }
          }
        }
        frame 5 {
          n93 = Unbundle By Name(w273) -> ("SerialFormat"=w272:T3)
          n94 = case shown="Default" w272 {
            selector: w272 -> [_ w282]
            tunnel: w277 -> [w280 w295]
            tunnel: w276 -> [w278 w294]
            tunnel: w275 -> [_ w293]
            tunnel: [w280 w285] -> w274
            tunnel: w271 -> [w279 w290]
            tunnel: [w279 w289] -> w270
            tunnel: w269 -> [_ w288]
            tunnel: [w278 w284] -> w268
            tunnel: [_ TRUE] -> w267
            frame "" {
            }
            frame Default {
              n95 = call "Translator.Translate.Status (NoError).vi"("msg"=w288) -> ("Translated Msg"=w287:string)  [unwired: 10 in]
              n96 = Format Into String(w282) -> (resulting string=w281:string)  [unwired: 3 in, 1 out]
              n97 = Concatenate Strings(w287, w281) -> (w286:string)
              n98 = invoke on="Invoke Node" class="Tree (strict)" method="Edit Tree Items.Add Item to End"(reference=w294, error in=w295, "Left Cell"=w286, "Child Tag"=w293, "Item Indent"=1 ("New Item Indentation"), "Child Only?"=TRUE) -> (reference out=w284:refnum<vi>, error out=w285:errorcluster)  [unwired: 2 in, 6 out]
              n99 = Increment(x=w290) -> (x+1=w289:i32)
            }
          }
        }
        frame 6 {
          n100 = Unbundle By Name(w305) -> ("Err"=w304:errorcluster)
          n101 = case shown="Error" w304 {
            selector: w304 -> [_ w326]
            tunnel: w306 -> [_ w327]
            tunnel: w298 -> [w308 w321]
            tunnel: [w308 w320] -> w303
            tunnel: w302 -> [w309 w316]
            tunnel: [w309 w311] -> w301
            tunnel: w300 -> [_ w314]
            tunnel: w299 -> [w307 w313]
            tunnel: [w307 w312] -> w297
            tunnel: [_ TRUE] -> w296
            frame No Error {
            }
            frame Error {
              n102 = Unbundle(w326) -> ("code"=w325:i32, "source"=w323:string)  [unwired: 1 out]
              n103 = To Variant(anything=w325) -> (Variant=w324:variant)
              n104 = Build Array(w324, w323) -> (w322:variant[])
              n105 = call "Translator.Translate.Status (NoError).vi"("Arguments"=w322, "msg"=w327) -> ("Translated Msg"=w315:string)  [unwired: 9 in]
              n106 = Build Array(w315) -> (w319:string[])
              n107 = invoke on="Invoke Node" class="Tree (strict)" method="Edit Tree Items.Add Item to End"(reference=w313, error in=w316, "Child Text"=w319, "Child Tag"=w314, "Item Indent"=1 ("New Item Indentation"), "Child Only?"=TRUE) -> (reference out=w312:refnum<vi>, error out=w311:errorcluster)  [unwired: 2 in, 6 out]
              n108 = Increment(x=w321) -> (x+1=w320:i32)
            }
          }
        }
      }
      n109 = case shown="True" w130 {
        tunnel: w134 -> [_ w149]
        tunnel: w133 -> [_ w148]
        tunnel: w132 -> [w145 w147]
        tunnel: [w145 w146] -> w131
        frame False {
        }
        frame True {
          n110 = property on="Property Node" class="Tree (strict)"(reference=w148, error in=w147, "Active Item Row Number"=w149, "ActiveColNum"=-2 ("Active Cell:Active Column Number"), "CellBG"=u32 16777226, "CellFontColor"=u32 0, "CellFontSize"=u32 13 ("Active Cell:Cell Font:Size"), "Height"=15 ("Active Cell:Cell Size:Height")) -> (error out=w146:errorcluster)  [unwired: 1 out]
        }
      }
    }
    n111 = Compound Arithmetic op=ADD(w83, w85) -> (w82:i32)
  }
  "File content" <- w45
  n112 = call <vilib>:"Clear Errors.vi"("error in (no error)"=w52) -> ("error out"=w34:errorcluster)  [unwired: 5 in, 1 out]
  n113 = invoke on="Invoke Node" class="Tree (strict)" method="Open/Close.Open/Close All"(reference="File list tree", error in=w34, "Open"=FALSE ("Open?")) -> (reference out=w50:refnum<vi>, error out=w51:errorcluster)  [unwired: 1 in, 2 out]
  n114 = Index Array(array=w46) -> (element=w6:string)  [unwired: 1 in]
  n115 = Bundle By Name(cluster=T8 {"Node"="", "Column"=0} ("Top Left Visible Cell"), "Node"=w6) -> (w55:T8)
  n116 = property class="Tree (strict)"(reference=w50, error in=w51, "Val(Sgnl)"=w6, "EditPos"=T9 {"Row"=-1, "Column"=-1} ("Edit Position"), "TopLeft"=w55, "Allow Editing Cells"=w54, "AllowDragOutsideControl"=w54, "Allow Item Drag"=w54, "Allow Dragging of Parent Items"=w54, "Allow Drop"=w54, "Allow Dragging Between Items"=w54) -> (error out=w15:errorcluster)  [unwired: 1 out]
  n117 = call "Wait.Gui.Close.vi"("error in (no error)"=w15) -> ("error out"=→"error out":errorcluster)  [unwired: 10 in]
